vi "SendListFGV.vi"(7 "Set":bool, 9 "Data":string, 10 "アドレス":string, 11 "Send List":cluster{"Address":string, "Data":string}[](array[cluster])) -> (2 "空?":bool, 3 "Send List Out":cluster{"Address":string, "Data":string}[](array[cluster]), 4 "Send Log":cluster{"アドレス":string, "Data":string}[](array[cluster]))   [LabVIEW 2017]
doc: "送信するデータと、送り先のアドレスのクラスターのリストを保持します。\nこのリストに登録することでTCPでデータを送付します。"
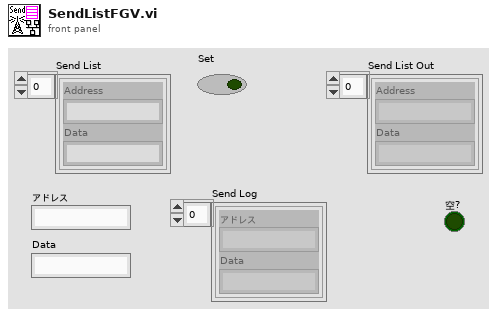
[diagram p1: front panel]
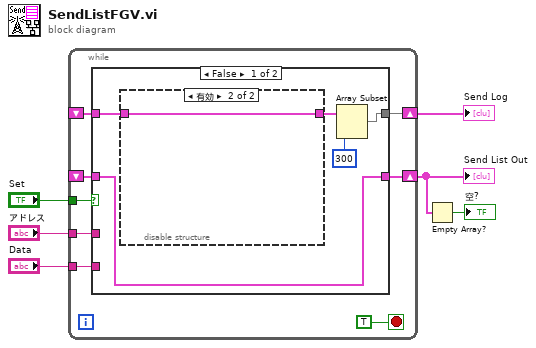
[diagram p0: block diagram]
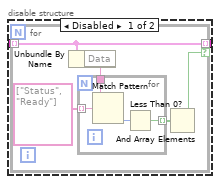
[diagram p2: hidden frame]
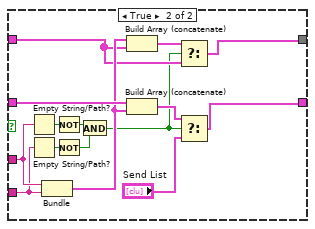
[diagram p3: hidden frame]
diagram:
  n1 = while {
    tunnel: "アドレス" -> [w12]
    tunnel: "Data" -> [w11]
    shift-right: [w14] -> w5
    shift-left: _ -> [w13]
    tunnel: "Set" -> [w9]
    shift-right: [w8] -> w1
    shift-left: _ -> [w7]
    stop <- TRUE stop-if-true
    n2 = case shown="FALSE" w9 {
      tunnel: [w19 w44] -> w14
      tunnel: w13 -> [w19 w46]
      tunnel: w12 -> [_ w42]
      tunnel: w11 -> [_ w39]
      tunnel: [w17 w34] -> w8
      tunnel: w7 -> [w16 w33]
      frame False {
        n3 = disable-structure shown="有効" {
          disable-tunnel: w16 -> [w21 w31]
          disable-tunnel: [w20 w31] -> w15
          frame Disabled {
            n4 = for {
              tunnel: w21 -> [w26] mode=indexing
              tunnel: [w26] -> w20 mode=indexing if=w22
              n5 = Unbundle By Name(w26) -> ("Data"=w24:string)
              n6 = for {
                tunnel: w24 -> [w30]
                tunnel: string[] ["Status", "Ready"] ("正規表現") -> [w29] mode=indexing
                tunnel: [w27] -> w23 mode=indexing
                n7 = Match Pattern(string=w30, regular expression=w29) -> (offset past match=w28:i32)  [unwired: 1 in, 3 out]
                n8 = Less Than 0?(x=w28) -> (x < 0?=w27:bool)
              }
              n9 = And Array Elements(Boolean array=w23) -> (logical AND=w22:bool)
            }
          }
          frame Enabled {
          }
        }
        n10 = Array Subset(array=w15, length=300 ("長さ")) -> (w17:cluster{"アドレス":string, "Data":string}[])  [unwired: 1 in]
      }
      frame True {
        n11 = Empty String/Path?(string/path=w42) -> (empty?=w41:bool)
        n12 = Empty String/Path?(string/path=w39) -> (empty?=w38:bool)
        n13 = Bundle("アドレス"=w42, "Data"=w39) -> (w36:cluster{"アドレス":string, "Data":string})  [unwired: 1 in]
        n14 = Not(x=w41) -> (.not. x?=w40:bool)
        n15 = Not(x=w38) -> (.not. x?=w37:bool)
        n16 = And(x=w40, y=w37) -> (x .and. y?=w32:bool)
        n17 = Build Array (concatenate)(w36, w33) -> (w35:cluster{"アドレス":string, "Data":string}[])
        n18 = Build Array (concatenate)(w46, w36) -> (w45:cluster{"アドレス":string, "Data":string}[])
        n19 = Select(t=w35, s=w32, f=w33) -> (s? t:f=w34:cluster{"アドレス":string, "Data":string}[])
        n20 = Select(t=w45, s=w32, f="Send List") -> (s? t:f=w44:cluster{"Address":string, "Data":string}[])
      }
    }
  }
  "Send List Out" <- w5
  "Send Log" <- w1
  n21 = Empty Array?(array=w5) -> (empty?=→"空?":bool)
